vi "GettingStarted_ComplexSignals.vi"() -> ()   [LabVIEW 2009]
uses:
  <vilib>/imath/engines/lvmath2/RunTimeEngine/ErrorHandling/NIMS_Finalize Error.vi
  <vilib>/imath/engines/lvmath2/RunTimeEngine/Parser/MC_Version.vi
  <vilib>/imath/engines/lvmath2/RunTimeEngine/NodeEndStatement/NIMS_NodeEndStatement_Output.vi
  <instcachedir>/0/NIMS_NodeEndStatement_Output_53EC0D466D134D7ABD903AC30B43404B.lvgen/NIMS_NodeEndStatement_Output_53EC0D466D134D7ABD903AC30B43404B_001.vi
  <vilib>/imath/engines/lvmath2/RunTimeEngine/RangeToken/NIMS_Range.vi
  <instcachedir>/0/NIMS_Range_08574DECC23E450FAF0AC0BC39E6BEA7.lvgen/NIMS_Range_08574DECC23E450FAF0AC0BC39E6BEA7_001.vi
  <vilib>/imathl/engines/lvmath/Functions/Error Handling/Create Error.vi
  <vilib>/imath/engines/lvmath2/RunTimeEngine/ArithmeticOperatorToken/NIMS_ArithmeticOperator_plus.vi
  <instcachedir>/0/NIMS_ArithmeticOperator_plus_48B9519178ED42D7840F01273E784BFE.lvgen/NIMS_ArithmeticOperator_plus_48B9519178ED42D7840F01273E784BFE_001.vi
  <vilib>/imath/engines/lvmath/Functions/Error Handling/MC_Error Cluster From Error Code.vi
  <vilib>/imath/engines/lvmath2/RunTimeEngine/BuiltInFunctions/rand/NIMS_rand(1,I32).vi
  <instcachedir>/0/NIMS_ArithmeticOperator_plus_48B9519178ED42D7840F01273E784BFE.lvgen/NIMS_ArithmeticOperator_plus_48B9519178ED42D7840F01273E784BFE_002.vi
  <vilib>/imath/engines/lvmath/Functions/Error Handling/MergeErrorsWrapper.vi
  <vilib>/imath/engines/lvmath2/RunTimeEngine/BuiltInFunctions/abs/NIMS_abs(signed).vi
  <instcachedir>/0/NIMS_abs(signed)_C4FCB8E6058B49B797C7C8D53CA5F6EC.lvgen/NIMS_abs(signed)_C4FCB8E6058B49B797C7C8D53CA5F6EC_000.vi
  <vilib>/imath/engines/lvmath2/RunTimeEngine/BuiltInFunctions/fft/NIMS_fft(GV).vi
  <instcachedir>/0/NIMS_fft(GV)_4C6467FC22F84E4BA42517A07EF978B0.lvgen/NIMS_fft(GV)_4C6467FC22F84E4BA42517A07EF978B0_000.vi
panel:
  out "Signal+noise (Frequency Domain)":dbl[](graph)
  out "x":dbl[](graph)
  out "noise (Time Domain)":dbl[](graph)
  in  "np":dbl=64.0 caption="Number of Points"
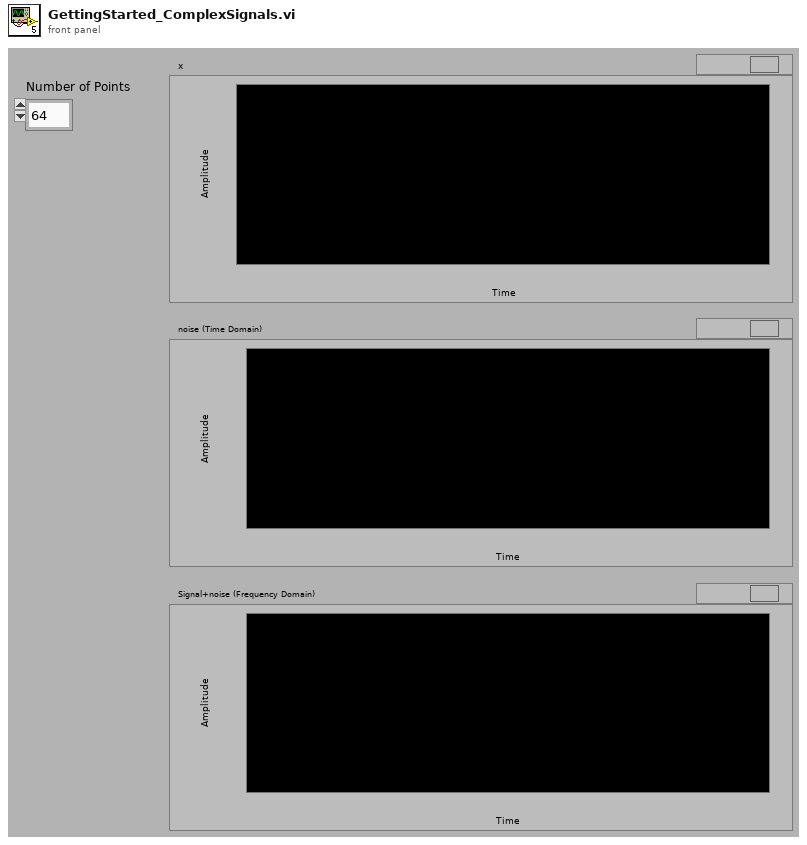
[diagram p1: front panel]
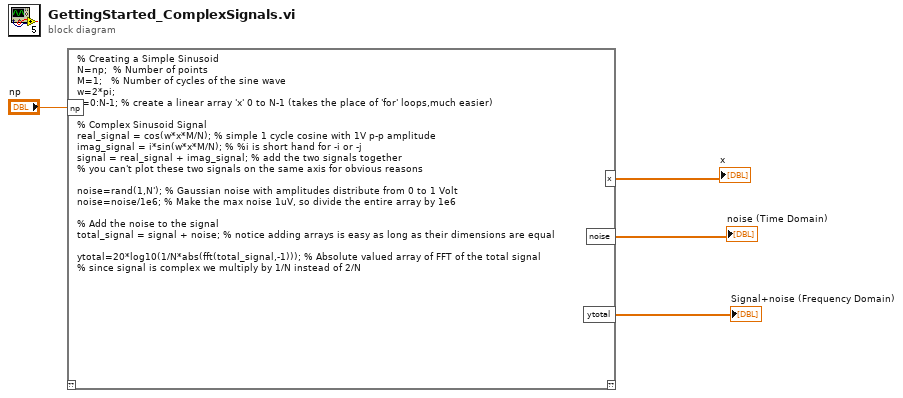
[diagram p0: block diagram]
diagram:
  n1 = mathscript code="% Creating a Simple Sinusoid\nN=np;  % Number of points\nM=1;   % Number of cycles of the sine wave\nw=2*pi; \nx=0:N-1; % create a linear array 'x' 0 to N-1 (takes the place of 'for' loops,much easier)\n\n% Complex Sinusoid Signal\nreal_signal = cos(w*x*M/N); % simple 1 cycle cosine with 1V p-p amplitude\nimag_signal = i*sin(w*x*M/N); % %i is short hand for -i or -j\nsignal = real_signal + imag_signal; % add the two signals together\n% you can't plot these two signals on the same axis for obvious reasons\n\nnoise=rand(1,N'); % Gaussian noise with amplitudes distribute from 0 to 1 Volt\nnoise=noise/1e6; % Make the max noise 1uV, so divide the entire array by 1e6\n\n% Add the noise to the signal\ntotal_signal = signal + noise; % notice adding arrays is easy as long as their dimensions are equal\n\nytotal=20*log10(1/N*abs(fft(total_signal,-1))); % Absolute valued array of FFT of the total signal \n% since signal is complex we multiply by 1/N instead of 2/N"("np"="np") -> ("noise"=→"noise (Time Domain)":dbl[], "ytotal"=→"Signal+noise (Frequency Domain)":dbl[], "x"=→"x":dbl[])  [unwired: 1 in, 1 out]
